vi "Get Incoming Single Point Settings.vi"(8 "error in":errorcluster, 10 "database in":refnum<k21>, 11 "Item Ref":T1 format="%.0x") -> (0 "error out":errorcluster, 1 "Incoming Single Point Configuraiton":T3, 2 "database out":refnum<k21>, 3 "Item Ref out":T1 format="%.0x", 4 "# of Channels":u32, 6 "Refs":T2 {"VS Refs" format="%.0x"})   [LabVIEW 2015, in "J1939 Addon System Explorer.lvlib"]
uses:
  J1939 Addon System Explorer.lvlib
  <vilib>/NI Veristand/Custom Device API/Custom Device Item Ref.ctl
  Shared/Types/SysDef Incoming Single Point Configurations.ctl
  Shared/Types/SysDef Incoming Frame Configuration.ctl
  Shared/Types/Incoming Single Point Channel Pairs.ctl
  <vilib>/NI Veristand/Custom Device API/Get Item Property (U32).vi
  <vilib>/NI Veristand/Custom Device Tools/Custom Device Utility Library/NI VeriStand - Search for All Items by GUID.vi
  Shared/SubVIs/Constants.vi
  <vilib>/NI VeriStand/Custom Device API/Custom Device API.lvlib
  Shared/J1939 Addon Shared.lvlib
  <resource>/objmgr/xnet.rc
  <vilib>/NI Veristand/Custom Device Tools/Custom Device Utility Library/Custom Device Utility Library.lvlib
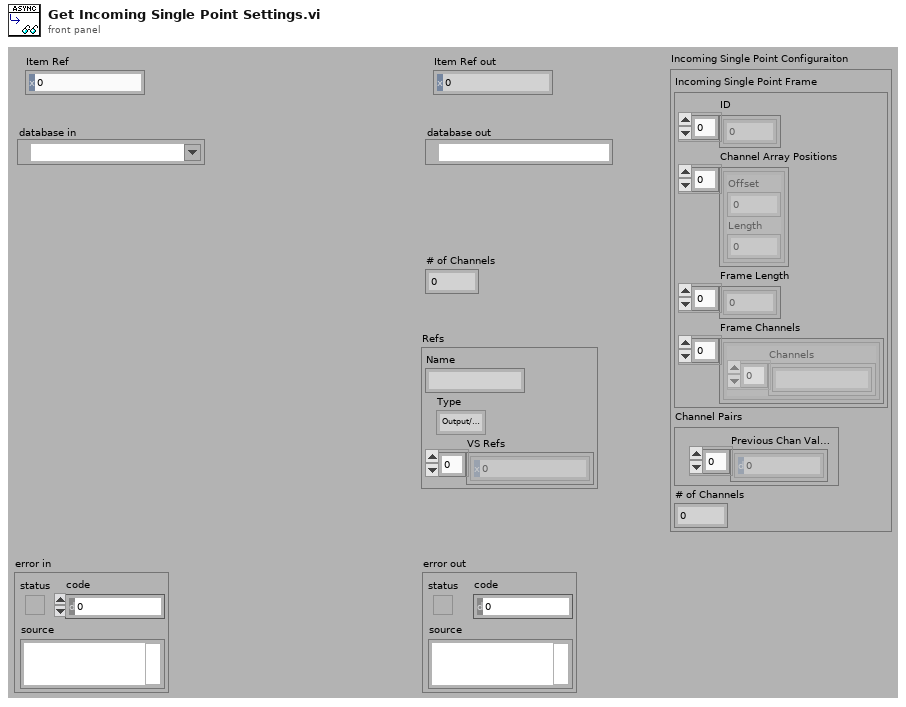
[diagram p1: front panel]
types:
  T1 = typedef "Custom Device API.lvlib/Custom Device Item Ref.ctl" = u64
  T2 = cluster{"Name":string, "Type":enum16{"Output/Write", "Input/Read", "Input/ReadWrite"}, "VS Refs":T1[]}
  T3 = typedef "J1939 Addon Shared.lvlib/SysDef Incoming Single Point Configurations.ctl" = cluster{"Incoming Single Point Frame":T4, "Channel Pairs":T5, "# of Channels":u32}
  T4 = typedef "J1939 Addon Shared.lvlib/SysDef Incoming Frame Configuration.ctl" = cluster{"ID":u32[], "Channel Array Positions":cluster{"Offset":u32, "Length":u32}[], "Frame Length":u32[], "Frame Channels":cluster{"Channels":string[]}[]}
  T5 = typedef "J1939 Addon Shared.lvlib/Incoming Single Point Channel Pairs.ctl" = cluster{"Previous Chan Values":dbl[]}
  T6 = enum16{"Output/Write", "Input/Read", "Input/ReadWrite"}
  T7 = typedef "Custom Device API.lvlib/Custom Device Item Info.ctl" = cluster{"Name":string, "Is Channel":bool, "GUID":string, "Is Waveform":bool}
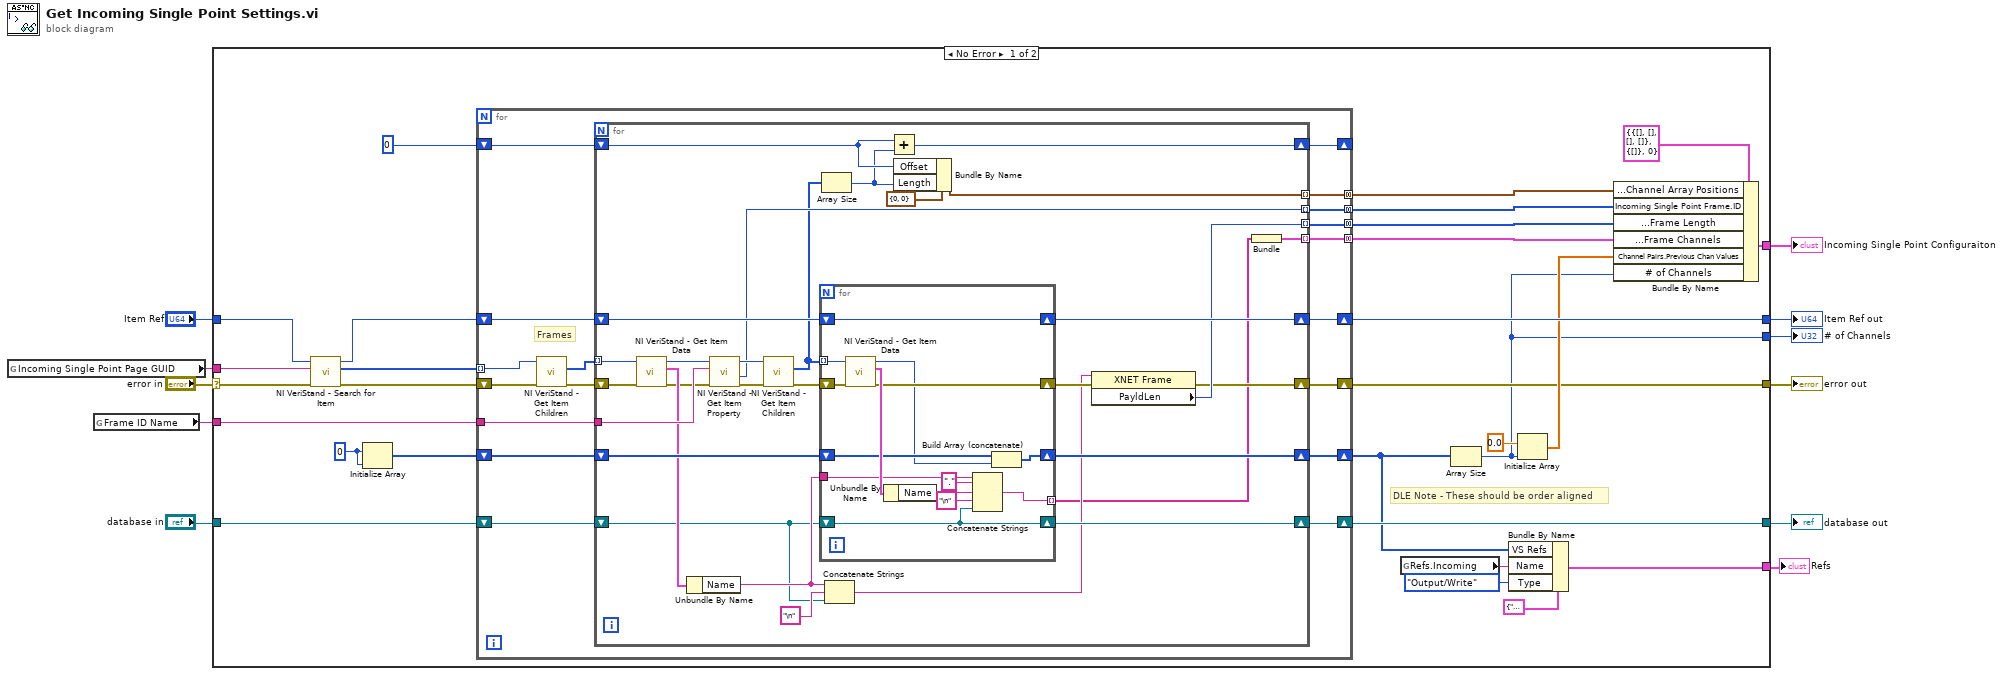
[diagram p0: block diagram]
diagram:
  n1 = global read "Constants.vi" "Incoming Single Point Page GUID"() -> (w6:string)
  n2 = global read "Constants.vi" "Frame ID Name"() -> (w9:string)
  n3 = case shown="No Error" "error in" {
    selector: "error in" -> [w21 w103]
    tunnel: "database in" -> [w26 w104]
    tunnel: [w35 w102] -> w10
    tunnel: [w31 _] -> w3
    tunnel: w9 -> [w39 _]
    tunnel: [w24 w103] -> w8
    tunnel: "Item Ref" -> [w19 w102]
    tunnel: w6 -> [w20 _]
    tunnel: [w36 w104] -> w5
    tunnel: [w22 _] -> w2
    tunnel: [w12 _] -> w1
    frame No Error {
      w13 = T1 0 ("Item Ref out")
      # "DLE Note - These should be order aligned"
      n4 = call-poly <vilib>:"NI VeriStand - Search for Item.vi"("error in"=w21, "Item GUID"=w20, "Section Ref in"=w19) -> ("error out"=w38:errorcluster, "Item Refs"=w37:T1[], "Section Ref out"=w18:T1)  [unwired: 5 in, 1 out]
      n5 = Initialize Array(w13, w13) -> (w34:T1[])
      n6 = for {
        tunnel: w39 -> [w57]
        tunnel: w37 -> [w54] mode=indexing
        tunnel: [w50] -> w30 mode=concatenating
        tunnel: [w47] -> w28 mode=concatenating
        tunnel: [w44] -> w25 mode=concatenating
        tunnel: [w42] -> w23 mode=concatenating
        shift-right: [w49] -> w14
        shift-left: w34 -> [w51]
        shift-right: [w53] -> w36
        shift-left: w26 -> [w46]
        shift-right: [w52] -> w35
        shift-left: w18 -> [w41]
        shift-right: [w43] -> w24
        shift-left: w38 -> [w55]
        shift-right: [w40] -> _
        shift-left: u32 0 -> [w48]
        # "Frames"
        n7 = call <vilib>:"NI VeriStand - Get Item Children.vi"("error in (no error)"=w55, "Item Ref in"=w54) -> ("error out"=w45:errorcluster, "Child Refs"=w56:T1[])  [unwired: 6 in, 2 out]
        n8 = for {
          shift-right: [w60] -> w43
          shift-left: w45 -> [w70]
          tunnel: w56 -> [w71] mode=indexing
          tunnel: w57 -> [w87]
          shift-right: [w84] -> w53
          shift-left: w46 -> [w63]
          shift-right: [w81] -> w52
          shift-left: w41 -> [w82]
          shift-right: [w79] -> w49
          shift-left: w51 -> [w80]
          tunnel: [w78] -> w50 mode=indexing
          shift-right: [w76] -> w40
          shift-left: w48 -> [w74]
          tunnel: [w72] -> w47 mode=indexing
          tunnel: [w68] -> w44 mode=indexing
          tunnel: [w58] -> w42 mode=indexing
          n9 = call <vilib>:"NI VeriStand - Get Item Data.vi"("error in (no error)"=w70, "Item Ref in"=w71) -> ("error out"=w66:errorcluster, "Item Info"=w69:T7, "Item Ref out"=w67:T1)  [unwired: 6 in, 1 out]
          n10 = Unbundle By Name(w69) -> ("Name"=w64:string)
          n11 = call-poly <vilib>:"NI VeriStand - Get Item Property.vi"("error in (no error)"=w66, "Property Name"=w87, "Item Ref in"=w67) -> ("error out"=w86:errorcluster, "Value"=w78:u32, "Item Ref out"=w85:T1)  [unwired: 5 in, 1 out]
          n12 = call <vilib>:"NI VeriStand - Get Item Children.vi"("error in (no error)"=w86, "Item Ref in"=w85) -> ("error out"=w83:errorcluster, "Child Refs"=w77:T1[])  [unwired: 6 in, 2 out]
          n13 = for {
            shift-right: [w90] -> w62
            shift-left: w83 -> [w100]
            tunnel: w77 -> [w101] mode=indexing
            tunnel: [w96] -> w59 mode=indexing
            shift-right: [w95] -> w84
            shift-left: w63 -> [w95]
            shift-right: [w88] -> w81
            shift-left: w82 -> [w88]
            shift-right: [w93] -> w79
            shift-left: w80 -> [w94]
            tunnel: w64 -> [w92]
            n14 = call <vilib>:"NI VeriStand - Get Item Data.vi"("error in (no error)"=w100, "Item Ref in"=w101) -> ("error out"=w90:errorcluster, "Item Info"=w99:T7, "Item Ref out"=w89:T1)  [unwired: 6 in, 1 out]
            n15 = Unbundle By Name(w99) -> ("Name"=w98:string)
            n16 = Concatenate Strings(w92, "." ("string"), w98, "\n" ("string"), w95) -> (w96:string)
            n17 = Build Array (concatenate)(w94, w89) -> (w93:T1[])
          }
          n18 = Array Size(array=w77) -> (size(s)=w73:i32)
          n19 = Concatenate Strings(w64, "\n" ("string"), w63) -> (w61:string)
          n20 = Add(x=w74, y=w73) -> (x+y=w76:u32)
          n21 = Bundle By Name(cluster=cluster{"Offset":u32, "Length":u32} {"Offset"=0, "Length"=0} ("Channel Array Position"), "Offset"=w74, "Length"=w73) -> (w72:cluster{"Offset":u32, "Length":u32})
          n22 = property class="XNET Frame"(reference=w61, error in=w62) -> (error out=w60:errorcluster, "PayldLen"=w68:u32)  [unwired: 1 out]
          n23 = Bundle(w59) -> (w58:cluster{string[]})  [unwired: 1 in]
        }
      }
      n24 = global read "Constants.vi" "Refs.Incoming"() -> (w16:string)
      n25 = Array Size(array=w14) -> (size(s)=w22:i32)
      n26 = Bundle By Name(cluster=T2 {"Name"="", "Type"=enum."Output/Write", "VS Refs"=[]} ("Group"), "VS Refs"=w14, "Name"=w16, "Type"=T6."Output/Write") -> (w12:T2)
      n27 = Initialize Array(0.0 ("element"), w22) -> (w27:dbl[])
      n28 = Bundle By Name(cluster=T3 {"Incoming Single Point Frame"={"ID"=[], "Channel Array Positions"=[], "Frame Length"=[], "Frame Channels"=[]}, "Channel Pairs"={"Previous Chan Values"=[]}, "# of Channels"=0} ("Incoming Single Point Configuraiton"), "Incoming Single Point Frame.Channel Array Positions"=w28, "Incoming Single Point Frame.ID"=w30, "Incoming Single Point Frame.Frame Length"=w25, "Incoming Single Point Frame.Frame Channels"=w23, "Channel Pairs.Previous Chan Values"=w27, "# of Channels"=w22) -> (w31:T3)
    }
    frame Error {
    }
  }
  "error out" <- w8
  "database out" <- w5
  "Item Ref out" <- w10
  "Incoming Single Point Configuraiton" <- w3
  "# of Channels" <- w2
  "Refs" <- w1
